vi "Waveform.vi"() -> ()   [LabVIEW 2019]
uses:
  caf06215-dee3-48c9-a013-d6da2cfc7d91.vi
panel:
  in  "stop":bool
  out "Waveform Chart":i16(graph)
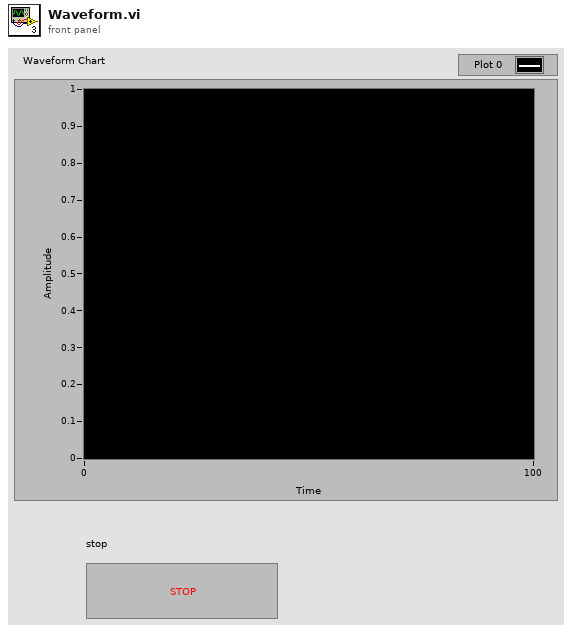
[diagram p1: front panel]
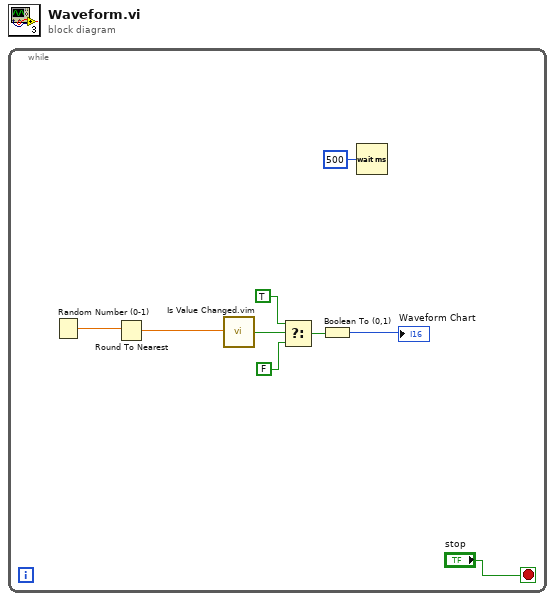
[diagram p0: block diagram]
diagram:
  n1 = while {
    stop <- "stop" stop-if-true
    n2 = Random Number (0-1)() -> (number: 0 to 1=w8:dbl)
    n3 = Round To Nearest(number=w8) -> (nearest integer value=w7:dbl)
    n4 = call "Is Value Changed.vim"("value"=w7) -> ("changed or first call?"=w6:bool)
    n5 = Select(t=TRUE, s=w6, f=FALSE) -> (s? t:f=w3:bool)
    n6 = Boolean To (0,1)(Boolean=w3) -> (0, 1=→"Waveform Chart":i16)
    n7 = Wait (ms)(milliseconds to wait=u32 500) -> ()  [unwired: 1 out]
  }
